vi "LED-SET.vi"(6 "Control_State":T1=enum."Solid", 7 "Numbers":dbl[](array[numeric])=[2.0, 4.0, 100.0, 30.0, 2.0, 6.0], 8 "colors":u32[](array[colorbox])=[16777215, 16777215, 16777215, 16777215, 16777215, 16777215, 16777215], 9 "Control_State 2":T1=enum."Solid", 10 "Control_State 3":T1=enum."Solid", 11 "Control_State 4":T1=enum."Solid") -> ()   [LabVIEW 2020]
uses:
  LED_Control_States.ctl
  LED GLOBALS!!!.vi
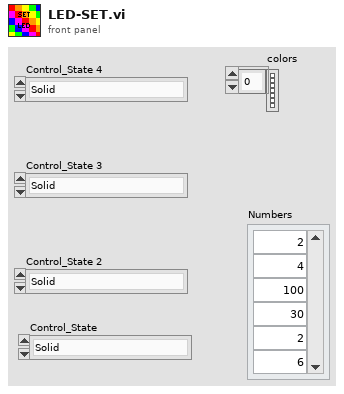
[diagram p1: front panel]
types:
  T1 = typedef "LED_Control_States.ctl" = enum16{"Config-Stripes", "swapperlines", "Rand", "Solid", "Flash-S", "Gradyent", "Move-Stripes", "Org-Rand", "Move-Point-Tail", "Flames", "Fade", "Alt-Colors"}
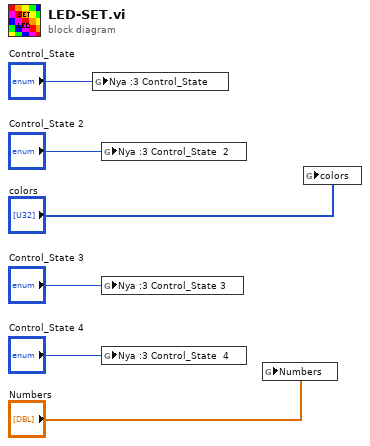
[diagram p0: block diagram]
diagram:
  n1 = global write "LED GLOBALS!!!.vi" "Nya :3 Control_State"("Control_State") -> ()
  n2 = global write "LED GLOBALS!!!.vi" "Nya :3 Control_State  2"("Control_State 2") -> ()
  n3 = global write "LED GLOBALS!!!.vi" "Nya :3 Control_State 3"("Control_State 3") -> ()
  n4 = global write "LED GLOBALS!!!.vi" "Nya :3 Control_State  4"("Control_State 4") -> ()
  n5 = global write "LED GLOBALS!!!.vi" "Numbers"("Numbers") -> ()
  n6 = global write "LED GLOBALS!!!.vi" "colors"("colors") -> ()
